vi "未命名 2.vi"() -> ()   [LabVIEW 2016]
panel:
  in  "大小":i32
  in  "数组元素.禁用":T1(ring)
  out "行数":u32
  in  "选择区域大小[]":u32[](array[numeric])
  in  "选择站点":bool[](array[boolean])
  out "行首字符串[]":string[](array[string])
  out "列首字符串[]":string[](array[string])
  out "information":T2(array[cluster])
  out "多列列表框":i32[](listbox)
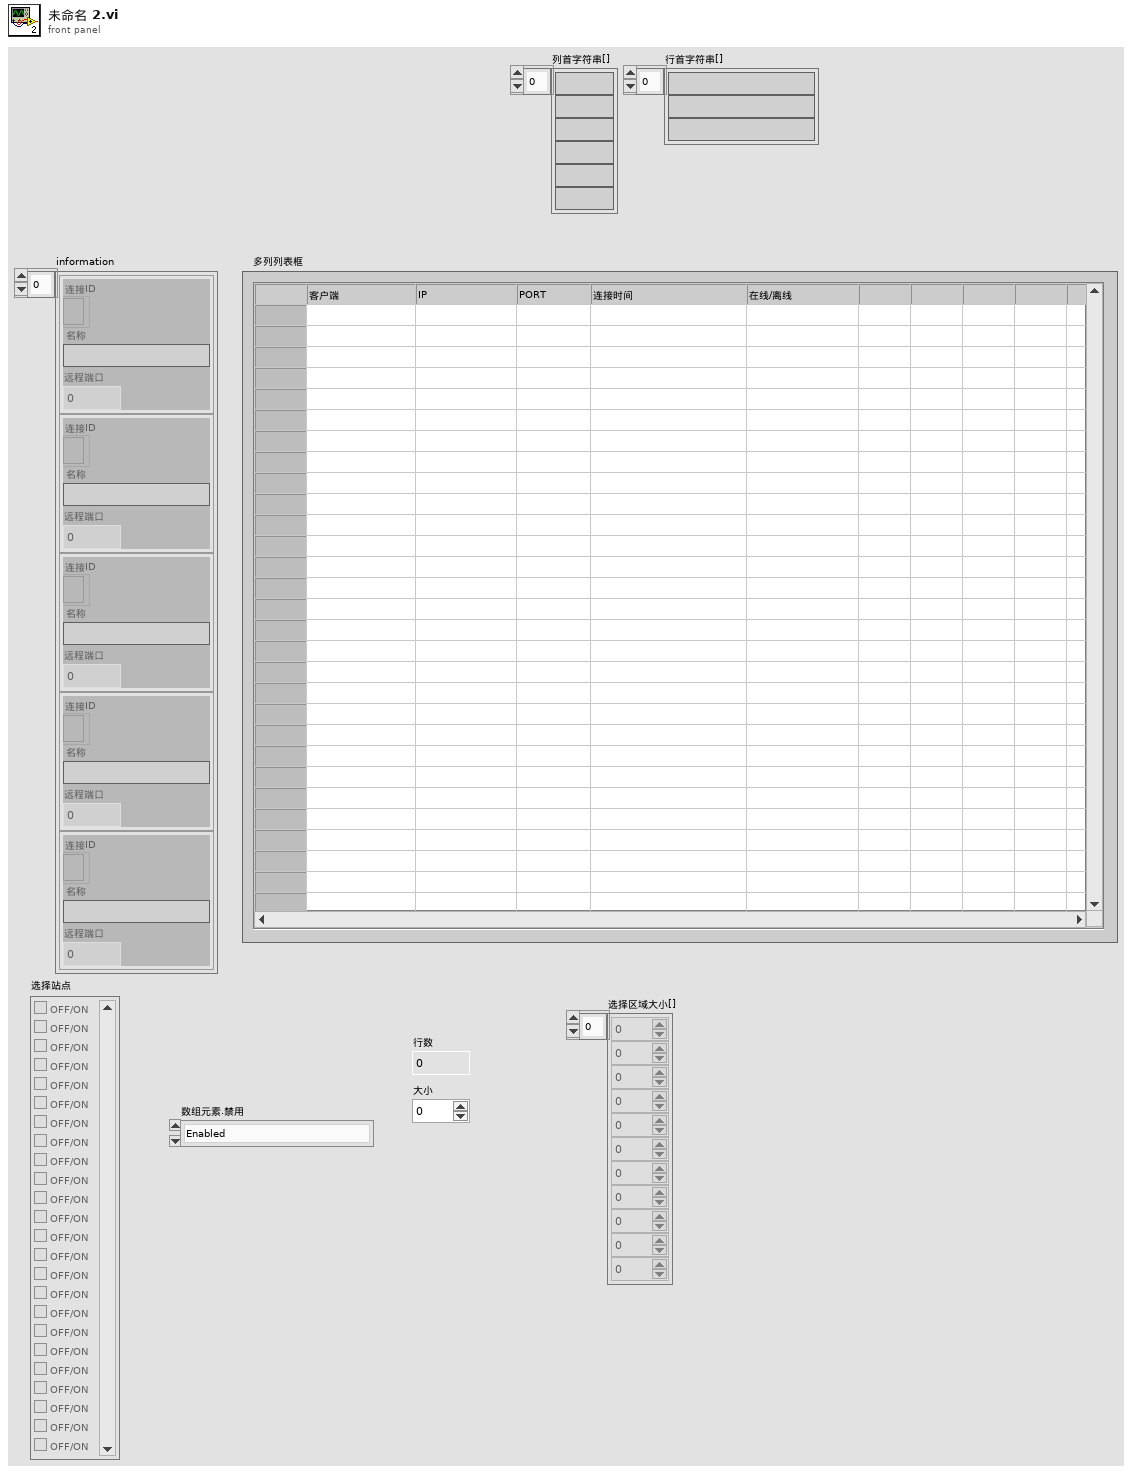
[diagram p1: front panel]
types:
  T1 = enum8{"Enabled", "Disabled", "Disabled and Grayed Out"}
  T2 = cluster{"连接ID":refnum<k5>, "名称":string, "远程端口":u16}[]
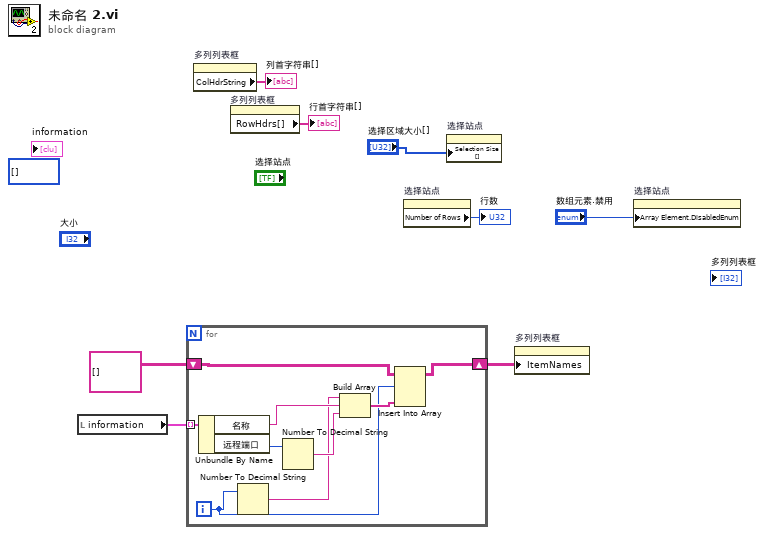
[diagram p0: block diagram]
diagram:
  (unwired) i32[] [] ("多列列表框")
  n1 = local read "information"() -> (w6:T2)
  n2 = for {
    tunnel: w6 -> [w17] mode=indexing
    shift-right: [w9] -> w4
    shift-left: string[][] [] ("项名") -> [w11]
    i -> [w10]
    n3 = Unbundle By Name(w17) -> ("名称"=w14:string, "远程端口"=w16:u16)
    n4 = Number To Decimal String(number=w10) -> (decimal integer string=w13:string)  [unwired: 1 in]
    n5 = Number To Decimal String(number=w16) -> (decimal integer string=w15:string)  [unwired: 1 in]
    n6 = Build Array(w13, w14, w15) -> (w12:string[])
    n7 = Insert Into Array(array=w11, index (row)=w10, new element=w12) -> (w9:string[][])  [unwired: 1 in]
  }
  n8 = property on="多列列表框" class="MCListbox (严格)"() -> ("ColHdrString"=→"列首字符串[]":string[])  [unwired: 2 in, 2 out]
  n9 = property on="多列列表框" class="MCListbox (严格)"() -> ("RowHdrs[]"=→"行首字符串[]":string[])  [unwired: 2 in, 2 out]
  n10 = property on="选择站点" class="Arr (严格)"() -> ("Number of Rows"=→"行数":u32)  [unwired: 2 in, 2 out]
  n11 = property on="选择站点" class="Arr (严格)"("Selection Size []"="选择区域大小[]") -> ()  [unwired: 2 in, 2 out]
  n12 = property on="多列列表框" class="MCListbox (严格)"("ItemNames"=w4) -> ()  [unwired: 2 in, 2 out]
  n13 = property on="选择站点" class="Arr (严格)"("Array Element.DisabledEnum"="数组元素.禁用") -> ()  [unwired: 2 in, 2 out]
